vi "Random.vi"(1 "Input 3":u8[][](array[numeric]), 4 "dimension size 2":i32, 5 "Input 2":u8[][](array[numeric]), 6 "dimension size":i32, 7 "seed":dbl, 9 "Input 1":u8[][](array[numeric]), 11 "Numeric":dbl) -> (0 "Output 3":u8[][](array[numeric]), 2 "Output 2":u8[][](array[numeric]), 3 "Output 1":u8[][](array[numeric]))   [LabVIEW 2016]
uses:
  <vilib>/Analysis/NI_AALBase.lvlib
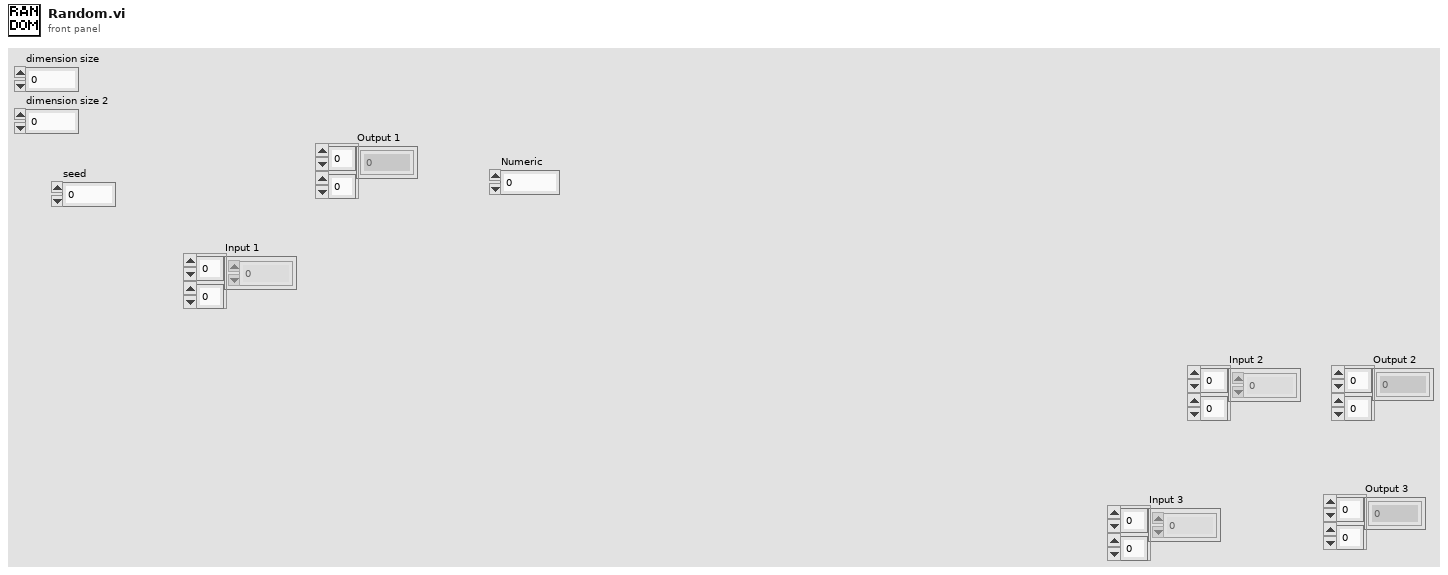
[diagram p1: front panel]
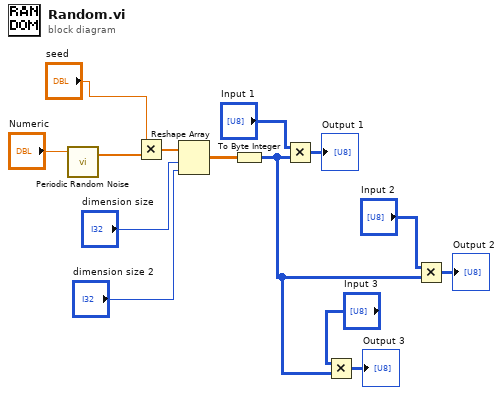
[diagram p0: block diagram]
diagram:
  n1 = call <vilib>:"Periodic Random Noise.vi"("samples"="Numeric") -> ("periodic random noise"=w10:dbl[])  [unwired: 2 in, 1 out]
  n2 = Multiply(x="seed", y=w10) -> (x*y=w11:dbl[])
  n3 = Reshape Array(w11, "dimension size", "dimension size 2") -> (w13:dbl[][])
  n4 = To Byte Integer(number=w13) -> (8bit integer=w1:i8[][])
  n5 = Multiply(x="Input 1", y=w1) -> (x*y=→"Output 1":u8[][])
  n6 = Multiply(x="Input 3", y=w1) -> (x*y=→"Output 3":u8[][])
  n7 = Multiply(x="Input 2", y=w1) -> (x*y=→"Output 2":u8[][])
